vi "Apply Column Setup After Binding.vi"(7 "DataTable":refnum<class "DataTable.lvclass">, 8 "error in (no error)":errorcluster, 11 "DataGridView in":refnum<class "DataGridView.lvclass">) -> (0 "error out":errorcluster, 3 "DataGridView out":refnum<class "DataGridView.lvclass">, 5 "DataTable out":refnum<class "DataTable.lvclass">)   [LabVIEW 2020, in "DataGrid.lvlib" / "DataGridView.lvclass"]
doc: "This is called after populating the datagridview (via binding its DataTable) so that the custom datatypes can be setup for the columns that require it. This is only needed if you are using <B>Buttons</B> or <B>Combos</B> as all other types are completely automatic."
uses:
  DataGridView.lvclass
  DataTable/DataTable.lvclass
  DataGridView.lvclass/DataGridView.ctl
  System.Windows.Forms
  GridColumn/GridColumn.lvclass/GridColumn.ctl
  GridColumn/Read Params.vi
  GridColumn/Read Caption.vi
  GridColumn/Read Name.vi
  GridColumn/Read AutoSizeMode.vi
  GridColumn/Read FillWeight.vi
  GridColumn/Read datatype.vi
  GridColumn/Read Tooltip.vi
  GridColumn/GridColumn.lvclass
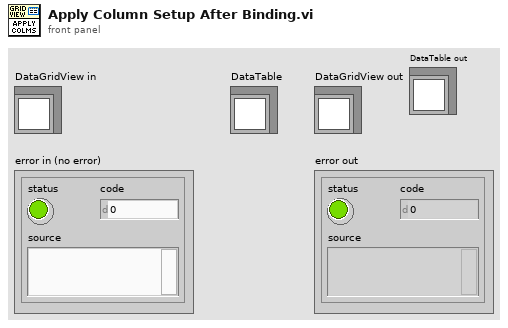
[diagram p1: front panel]
types:
  T1 = typedef "DataGrid.lvlib/GridColumn.lvclass/ColumnType.ctl" = enum16{"string", "image", "check", "numeric", "timestamp", "button", "combo", "link"}
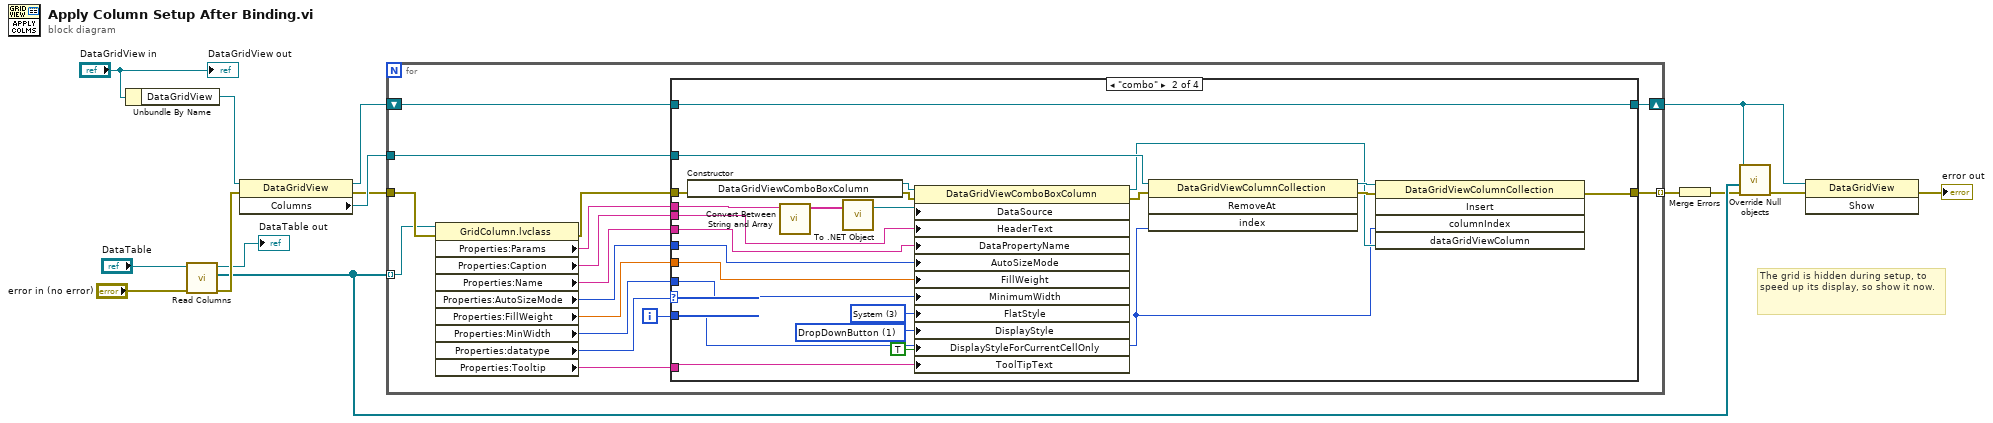
[diagram p0: block diagram]
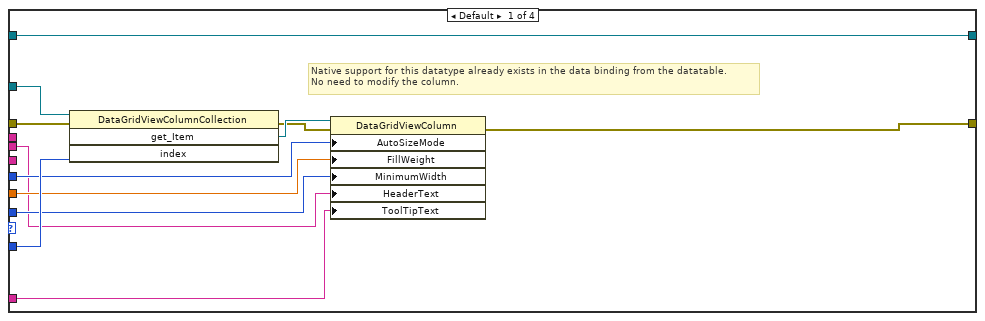
[diagram p2: hidden frame]
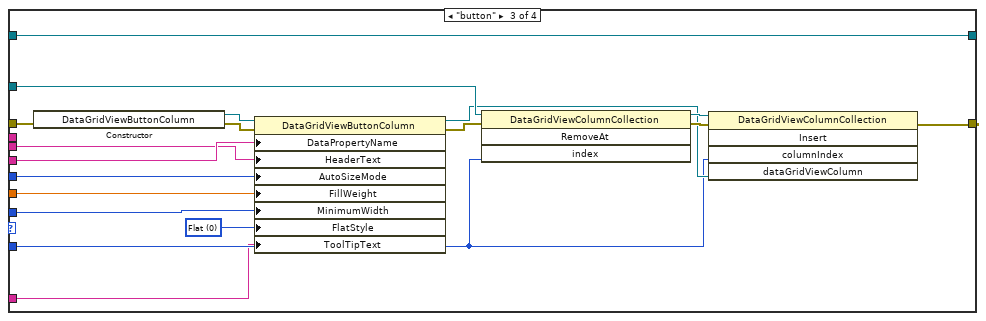
[diagram p3: hidden frame]
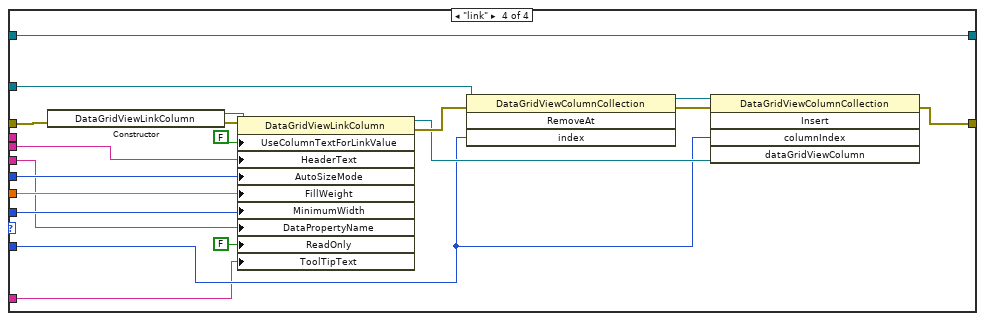
[diagram p4: hidden frame]
diagram:
  # "The grid is hidden during setup, to speed up its display, so show it now."
  n1 = Unbundle By Name("DataGridView in") -> ("DataGridView"=w13:refnum<k24>)
  n2 = call "Read Columns.vi"("error in (no error)"="error in (no error)", "DataTable in"="DataTable") -> ("error out"=w7:errorcluster, "Columns"=w6:refnum<class "GridColumn.lvclass">[], "DataTable out"=→"DataTable out":refnum<class "DataTable.lvclass">)  [unwired: 7 in]
  n3 = property class="DataGridView"(reference=w13, error in=w7) -> (reference out=w3:refnum<k24>, error out=w10:errorcluster, "Columns"=w12:refnum<k24>)
  n4 = for {
    tunnel: w12 -> [w31]
    tunnel: [w30] -> w14 mode=indexing
    tunnel: w10 -> [w21]
    tunnel: w6 -> [w20] mode=indexing
    shift-right: [w17] -> w2
    shift-left: w3 -> [w18]
    i -> [w29]
    n5 = property class="GridColumn.lvclass"(reference=w20, error in=w21) -> (error out=w22:errorcluster, "Properties:Params"=w28:string, "Properties:Caption"=w19:string, "Properties:Name"=w27:string, "Properties:AutoSizeMode"=w26:i32, "Properties:FillWeight"=w23:sgl, "Properties:MinWidth"=w25:i32, "Properties:datatype"=w24:T1, "Properties:Tooltip"=w16:string)  [unwired: 1 out]
    n6 = case shown="\"combo\"" w24 {
      tunnel: w31 -> [w43 w64 w82 w94]
      tunnel: [w35 w45 w68 w93] -> w30
      tunnel: w29 -> [w42 w46 w69 w87]
      tunnel: w27 -> [_ w51 w74 w90]
      tunnel: w28 -> [_ w54 _ _]
      tunnel: w25 -> [w37 w55 w78 w97]
      tunnel: w23 -> [w38 w56 w77 w98]
      tunnel: w26 -> [w39 w57 w76 w99]
      tunnel: w22 -> [w36 w53 w75 w103]
      tunnel: w19 -> [w34 w52 w73 w89]
      tunnel: w18 -> [w33 w50 w72 w88]
      tunnel: [w33 w50 w72 w88] -> w17
      tunnel: w16 -> [w32 w44 w67 w85]
      frame Default {
        # "Native support for this datatype already exists in the data binding from the datatable.\nNo need to modify the column."
        n7 = invoke class="DataGridViewColumnCollection" method="get_Item"(reference=w43, error in=w36, "index"=w42) -> (error out=w40:errorcluster, "get_Item"=w41:refnum<k24>)  [unwired: 1 in, 2 out]
        n8 = property class="DataGridViewColumn"(reference=w41, error in=w40, "AutoSizeMode"=w39, "FillWeight"=w38, "MinimumWidth"=w37, "HeaderText"=w34, "ToolTipText"=w32) -> (error out=w35:errorcluster)  [unwired: 1 out]
      }
      frame "combo" {
        w48 = 1 items=["ComboBox", "DropDownButton", "Nothing"] ("DisplayStyle")
        w49 = 3 items=["Flat", "Popup", "Standard", "System"] ("FlatStyle")
        n9 = constructor class="DataGridViewComboBoxColumn"(error in=w53) -> (reference out=w66:refnum<k24>, error out=w65:errorcluster)  [unwired: 2 in, 1 out]
        n10 = call "Convert Between String and Array.vi"("String"=w54) -> ("String Array"=w58:string[])  [unwired: 9 in, 1 out]
        n11 = call <vilib>:"To .NET Object.vi"("anything"=w58) -> (".NET object"=w60:refnum<k24>)  [unwired: 1 in, 1 out]
        n12 = property class="DataGridViewComboBoxColumn"(reference=w66, error in=w65, "DataSource"=w60, "HeaderText"=w52, "DataPropertyName"=w51, "AutoSizeMode"=w57, "FillWeight"=w56, "MinimumWidth"=w55, "FlatStyle"=w49, "DisplayStyle"=w48, "DisplayStyleForCurrentCellOnly"=TRUE, "ToolTipText"=w44) -> (reference out=w61:refnum<k24>, error out=w59:errorcluster)
        n13 = invoke class="DataGridViewColumnCollection" method="RemoveAt"(reference=w64, error in=w59, "index"=w46) -> (reference out=w62:refnum<k24>, error out=w63:errorcluster)  [unwired: 1 in, 2 out]
        n14 = invoke class="DataGridViewColumnCollection" method="Insert"(reference=w62, error in=w63, "columnIndex"=w46, "dataGridViewColumn"=w61) -> (error out=w45:errorcluster)  [unwired: 1 in, 4 out]
      }
      frame "button" {
        w71 = 0 items=["Flat", "Popup", "Standard", "System"] ("FlatStyle")
        n15 = constructor class="DataGridViewButtonColumn"(error in=w75) -> (reference out=w84:refnum<k24>, error out=w83:errorcluster)  [unwired: 2 in, 1 out]
        n16 = property class="DataGridViewButtonColumn"(reference=w84, error in=w83, "DataPropertyName"=w74, "HeaderText"=w73, "AutoSizeMode"=w76, "FillWeight"=w77, "MinimumWidth"=w78, "FlatStyle"=w71, "ToolTipText"=w67) -> (reference out=w70:refnum<k24>, error out=w79:errorcluster)
        n17 = invoke class="DataGridViewColumnCollection" method="RemoveAt"(reference=w82, error in=w79, "index"=w69) -> (reference out=w80:refnum<k24>, error out=w81:errorcluster)  [unwired: 1 in, 2 out]
        n18 = invoke class="DataGridViewColumnCollection" method="Insert"(reference=w80, error in=w81, "columnIndex"=w69, "dataGridViewColumn"=w70) -> (error out=w68:errorcluster)  [unwired: 1 in, 4 out]
      }
      frame "link" {
        n19 = constructor class="DataGridViewLinkColumn"(error in=w103) -> (reference out=w102:refnum<k24>, error out=w101:errorcluster)  [unwired: 2 in, 1 out]
        n20 = property class="DataGridViewLinkColumn"(reference=w102, error in=w101, "UseColumnTextForLinkValue"=FALSE, "HeaderText"=w89, "AutoSizeMode"=w99, "FillWeight"=w98, "MinimumWidth"=w97, "DataPropertyName"=w90, "ReadOnly"=FALSE, "ToolTipText"=w85) -> (reference out=w91:refnum<k24>, error out=w92:errorcluster)
        n21 = invoke class="DataGridViewColumnCollection" method="RemoveAt"(reference=w94, error in=w92, "index"=w87) -> (reference out=w95:refnum<k24>, error out=w96:errorcluster)  [unwired: 1 in, 2 out]
        n22 = invoke class="DataGridViewColumnCollection" method="Insert"(reference=w95, error in=w96, "columnIndex"=w87, "dataGridViewColumn"=w91) -> (error out=w93:errorcluster)  [unwired: 1 in, 4 out]
      }
    }
  }
  n23 = Merge Errors(w14) -> (w5:errorcluster)
  n24 = call "Override Null objects.vi"("error in (no error)"=w5, "Columns"=w6, ".NET Refnum in"=w2) -> ("error out"=w4:errorcluster)  [unwired: 8 in]
  n25 = invoke class="DataGridView" method="Show"(reference=w2, error in=w4) -> (error out=→"error out":errorcluster)  [unwired: 1 in, 2 out]
  "DataGridView out" <- "DataGridView in"
